vi "tool_Unicode_Display Ring Texts.vi"(5 "Interpret as Unicode (T)":bool, 6 "error in":errorcluster, 8 "Ring Texts":string[](array[string]), 9 "Ring Control Ref":refnum<vi>) -> (0 "error out":errorcluster, 3 "Ring Control Ref":refnum<vi>)   [LabVIEW 2009]
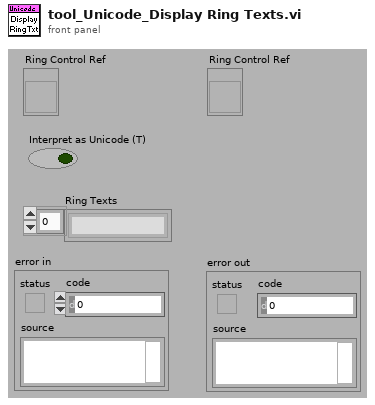
[diagram p1: front panel]
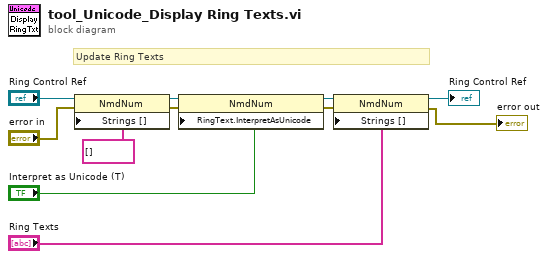
[diagram p0: block diagram]
diagram:
  # "Update Ring Texts"
  n1 = property class="NmdNum"(reference="Ring Control Ref", error in="error in", "Strings []"=string[] [] ("Strings [4]")) -> (reference out=w4:refnum<vi>, error out=w5:errorcluster)
  n2 = property class="NmdNum"(reference=w4, error in=w5, "RingText.InterpretAsUnicode"="Interpret as Unicode (T)") -> (reference out=w8:refnum<vi>, error out=w7:errorcluster)
  n3 = property class="NmdNum"(reference=w8, error in=w7, "Strings []"="Ring Texts") -> (reference out=→"Ring Control Ref":refnum<vi>, error out=→"error out":errorcluster)
